vi "重启.vi"(0 "Display State In":T1={"华氏?"=FALSE, "显示模式开关？"=TRUE}, 5 "重启":bool, 9 "Container State":T2, 11 "error in (no error)":errorcluster) -> (4 "Display State Out":T1={"华氏?"=FALSE, "显示模式开关？"=TRUE}, 15 "error out":errorcluster)   [LabVIEW 2011, in "双模温度计2.xctl"]
uses:
  <vilib>/_xctls/Container State.ctl
  State.ctl
  <vilib>/_xctls/XControlSupport.lvlib
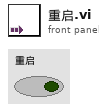
[diagram p1: front panel]
types:
  T1 = typedef "双模温度计2.xctl/State.ctl" = cluster{"华氏?":bool, "显示模式开关？":bool}
  T2 = typedef "XControlSupport.lvlib/Container State.ctl" = cluster{"Indicator?":bool, "Run Mode?":bool, " Refnum":refnum<vi>}
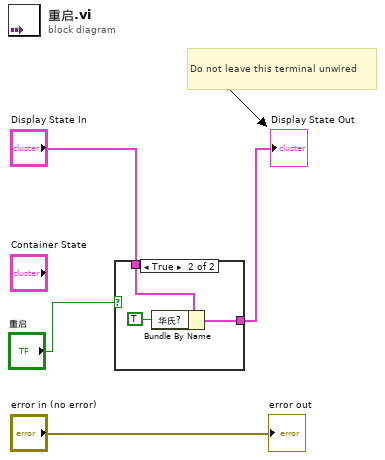
[diagram p0: block diagram]
diagram:
  # "Do not leave this terminal unwired"
  n1 = case shown="True" "重启" {
    tunnel: "Display State In" -> [w5 w8]
    tunnel: [w5 w6] -> w1
    frame False {
    }
    frame True {
      n2 = Bundle By Name(cluster=w8, "华氏?"=TRUE) -> (w6:T1)
    }
  }
  "Display State Out" <- w1
  "error out" <- "error in (no error)"
